vi "Get Steps from File.vi"(11 "Steps File":path) -> (0 "error out":errorcluster, 1 "Steps":i32, 2 "Table Steps":dbl[](array[numeric]), 3 "File Path out":path, 4 "End":dbl, 5 "Start":dbl)   [LabVIEW 2019, in "Acquisition Example.lvlib"]
uses:
  Acquisition Example.lvlib
  <vilib>/Utility/file.llb/Read Delimited Spreadsheet (DBL).vi
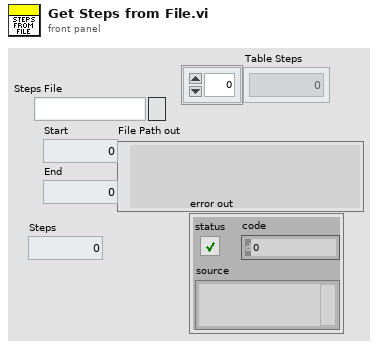
[diagram p1: front panel]
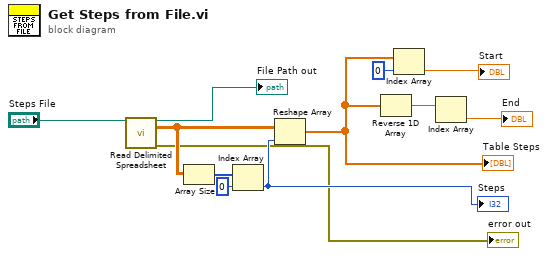
[diagram p0: block diagram]
diagram:
  n1 = call-poly <vilib>:"Read Delimited Spreadsheet.vi"("file path (dialog if empty)"="Steps File") -> ("new file path (Not A Path if cancelled)"=→"File Path out":path, "all rows"=w10:dbl[][], "error out"=→"error out":errorcluster)  [unwired: 9 in, 3 out]
  n2 = Array Size(array=w10) -> (size(s)=w11:i32[])
  n3 = Index Array(array=w11, index=0) -> (element=w2:i32)
  "Steps" <- w2
  n4 = Reshape Array(w10, w2) -> (w5:dbl[])
  "Table Steps" <- w5
  n5 = Reverse 1D Array(array=w5) -> (reversed array=w4:dbl[])
  n6 = Index Array(array=w5, index=0) -> (element=→"Start":dbl)
  n7 = Index Array(array=w4) -> (element=→"End":dbl)  [unwired: 1 in]
